vi "Set configuration chain.vi"(8 "error in (no error)":errorcluster, 9 "class names":string[](array[string]), 10 "configuration":variant[](array[variant]), 11 "Tomo in":refnum<class "Tomo.lvclass">) -> (0 "error out":errorcluster, 3 "Tomo out":refnum<class "Tomo.lvclass">)   [LabVIEW 2012, in "Tomo.lvclass"]
uses:
  Tomo.lvclass
  <vilib>/Distrio/Murmex/Murmex/Murmex.lvclass
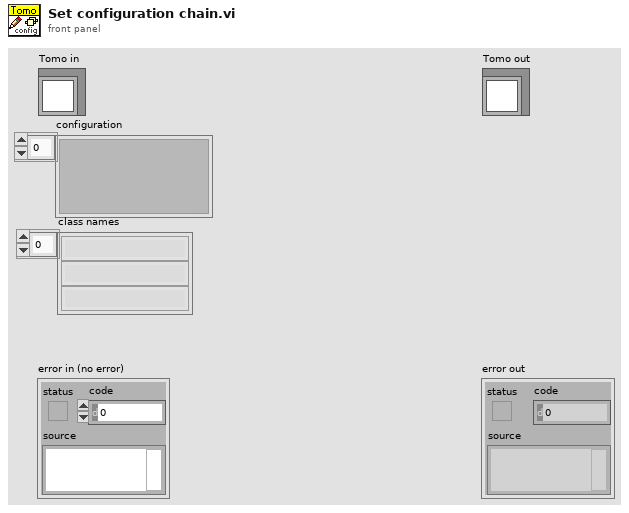
[diagram p1: front panel]
types:
  T1 = typedef "Tomo.lvclass/configuration cluster.ctl" = cluster{"stack component":string, "camera component":string, "stages component":string, "mapping file folder":path, "default stages speed":dbl[unit], "stack overhead time":dbl[unit], "autofocus component":string, "imaging component":string, "AOTF component":string}
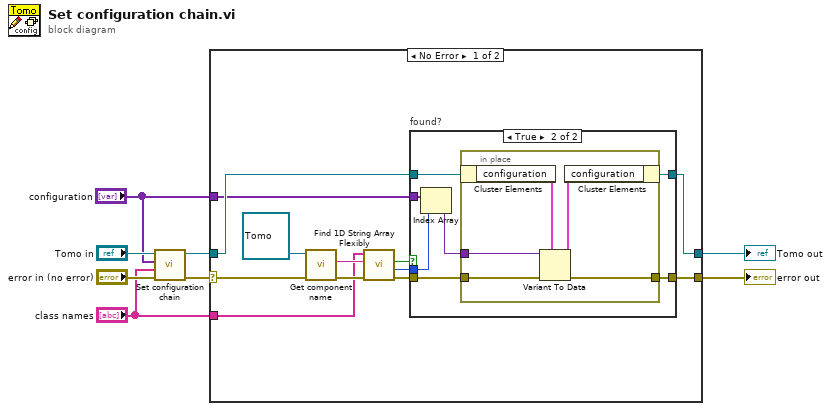
[diagram p0: block diagram]
diagram:
  n1 = call-parent "Set configuration chain.vi"("error in (no error)"="error in (no error)", "class names"="class names", "configuration"="configuration", "Murmex in"="Tomo in") -> ("error out"=w6:errorcluster, "Murmex out"=w3:refnum<class "Tomo.lvclass">)  [unwired: 6 in]
  n2 = case shown="No Error" w6 {
    selector: w6 -> [w11 w36]
    tunnel: [w15 w36] -> w5
    tunnel: [w9 w35] -> w4
    tunnel: w3 -> [w13 w35]
    tunnel: "class names" -> [w14 _]
    tunnel: "configuration" -> [w12 _]
    frame No Error {
      n3 = call <vilib>:"Get component name.vi"("error in (no error)"=w11, "Murmex in"=refnum<class "Tomo.lvclass"> refnum ("Tomo out")) -> ("error out"=w20:errorcluster, "component name"=w18:string)  [unwired: 7 in, 1 out]
      n4 = call <vilib>:"Find 1D String Array Flexibly.vi"("error in (no error)"=w20, "element"=w18, "array"=w14) -> ("error out"=w19:errorcluster, "index of element"=w17:i32, "found?"=w16:bool)  [unwired: 6 in]
      n5 = case "found?" shown="True" w16 {
        tunnel: w12 -> [_ w29]
        tunnel: w13 -> [w22 w27]
        tunnel: [w22 w26] -> w9
        tunnel: [w21 w25] -> w15
        tunnel: w19 -> [w21 w24]
        tunnel: w17 -> [_ w23]
        frame False {
        }
        frame True {
          n6 = Index Array(array=w29, index=w23) -> (element=w28:variant)
          n7 = in-place {
            in-place-border: w28 -> [w34]
            in-place-border: w24 -> [w32]
            in-place-border: [w30] -> w25
            n8 = in-place-cluster #1(w27) -> ("configuration"=w33:T1)
            n9 = Variant To Data(error in=w32, type=w33, Variant=w34) -> (data=w31:T1, error out=w30:errorcluster)
            n10 = in-place-cluster #1("configuration"=w31) -> (w26:refnum<class "Tomo.lvclass">)
          }
        }
      }
    }
    frame Error {
    }
  }
  "error out" <- w5
  "Tomo out" <- w4
